vi "Calc_Volume.vi"(11 "Bridge":fxp<+/-,32,-1>) -> (3 "Numeric":dbl)   [LabVIEW 2019]
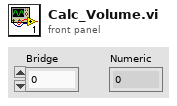
[diagram p1: front panel]
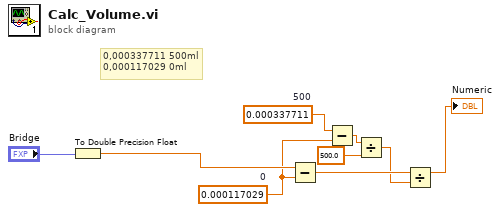
[diagram p0: block diagram]
diagram:
  w6 = 0.000337711  # 500
  w5 = 0.000117029  # 0
  # "0,000337711 500ml\n0,000117029 0ml"
  n1 = To Double Precision Float(number="Bridge") -> (double precision float=w9:dbl)
  n2 = Subtract(x=w9, y=w5) -> (x-y=w7:dbl)
  n3 = Subtract(x=w6, y=w5) -> (x-y=w4:dbl)
  n4 = Divide(x=w4, y=500.0) -> (x/y=w1:dbl)
  n5 = Divide(x=w7, y=w1) -> (x/y=→"Numeric":dbl)
